vi "FipsAdjacent.vi"() -> (11 "Fips":i32[](array[numeric]))   [LabVIEW 2017] (continued)
08079\t\"Hinsdale County, CO\"\t08053\n\"Mineral County, CO\"\t08079\t\"Mineral County, CO\"\t08079\n\"Mineral County, CO\"\t08079\t\"Rio Grande County, CO\"\t08105\n\"Mineral County, CO\"\t08079\t\"Saguache County, CO\"\t08109\n\"Moffat County, CO\"\t08081\t\"Moffat County, CO\"\t08081\n\"Moffat County, CO\"\t08081\t\"Rio Blanco County, CO\"\t08103\n\"Moffat County, CO\"\t08081\t\"Routt County, CO\"\t08107\n\"Moffat County, CO\"\t08081\t\"Daggett County, UT\"\t49009\n\"Moffat County, CO\"\t08081\t\"Uintah County, UT\"\t49047\n\"Moffat County, CO\"\t08081\t\"Carbon County, WY\"\t56007\n\"Moffat County, CO\"\t08081\t\"Sweetwater County, WY\"\t56037\n\"Montezuma County, CO\"\t08083\t\"Apache County, AZ\"\t04001\n\"Montezuma County, CO\"\t08083\t\"Dolores County, CO\"\t08033\n\"Montezuma County, CO\"\t08083\t\"La Plata County, CO\"\t08067\n\"Montezuma County, CO\"\t08083\t\"Montezuma County, CO\"\t08083\n\"Montezuma County, CO\"\t08083\t\"San Juan County, CO\"\t08111\n\"Montezuma County, CO\"\t08083\t\"San Juan County, NM\"\t35045\n\"Montezuma County, CO\"\t08083\t\"San Juan County, UT\"\t49037\n\"Montrose County, CO\"\t08085\t\"Delta County, CO\"\t08029\n\"Montrose County, CO\"\t08085\t\"Gunnison County, CO\"\t08051\n\"Montrose County, CO\"\t08085\t\"Mesa County, CO\"\t08077\n\"Montrose County, CO\"\t08085\t\"Montrose County, CO\"\t08085\n\"Montrose County, CO\"\t08085\t\"Ouray County, CO\"\t08091\n\"Montrose County, CO\"\t08085\t\"San Miguel County, CO\"\t08113\n\"Montrose County, CO\"\t08085\t\"Grand County, UT\"\t49019\n\"Montrose County, CO\"\t08085\t\"San Juan County, UT\"\t49037\n\"Morgan County, CO\"\t08087\t\"Adams County, CO\"\t08001\n\"Morgan County, CO\"\t08087\t\"Logan County, CO\"\t08075\n\"Morgan County, CO\"\t08087\t\"Morgan County, CO\"\t08087\n\"Morgan County, CO\"\t08087\t\"Washington County, CO\"\t08121\n\"Morgan County, CO\"\t08087\t\"Weld County, CO\"\t08123\n\"Otero County, CO\"\t08089\t\"Bent County, CO\"\t08011\n\"Otero County, CO\"\t08089\t\"Crowley County, CO\"\t08025\n\"Otero County, CO\"\t08089\t\"Kiowa County, CO\"\t08061\n\"Otero County, CO\"\t08089\t\"Las Animas County, CO\"\t08071\n\"Otero County, CO\"\t08089\t\"Otero County, CO\"\t08089\n\"Otero County, CO\"\t08089\t\"Pueblo County, CO\"\t08101\n\"Ouray County, CO\"\t08091\t\"Gunnison County, CO\"\t08051\n\"Ouray County, CO\"\t08091\t\"Hinsdale County, CO\"\t08053\n\"Ouray County, CO\"\t08091\t\"Montrose County, CO\"\t08085\n\"Ouray County, CO\"\t08091\t\"Ouray County, CO\"\t08091\n\"Ouray County, CO\"\t08091\t\"San Juan County, CO\"\t08111\n\"Ouray County, CO\"\t08091\t\"San Miguel County, CO\"\t08113\n\"Park County, CO\"\t08093\t\"Chaffee County, CO\"\t08015\n\"Park County, CO\"\t08093\t\"Clear Creek County, CO\"\t08019\n\"Park County, CO\"\t08093\t\"Fremont County, CO\"\t08043\n\"Park County, CO\"\t08093\t\"Jefferson County, CO\"\t08059\n\"Park County, CO\"\t08093\t\"Lake County, CO\"\t08065\n\"Park County, CO\"\t08093\t\"Park County, CO\"\t08093\n\"Park County, CO\"\t08093\t\"Summit County, CO\"\t08117\n\"Park County, CO\"\t08093\t\"Teller County, CO\"\t08119\n\"Phillips County, CO\"\t08095\t\"Logan County, CO\"\t08075\n\"Phillips County, CO\"\t08095\t\"Phillips County, CO\"\t08095\n\"Phillips County, CO\"\t08095\t\"Sedgwick County, CO\"\t08115\n\"Phillips County, CO\"\t08095\t\"Yuma County, CO\"\t08125\n\"Phillips County, CO\"\t08095\t\"Chase County, NE\"\t31029\n\"Phillips County, CO\"\t08095\t\"Perkins County, NE\"\t31135\n\"Pitkin County, CO\"\t08097\t\"Chaffee County, CO\"\t08015\n\"Pitkin County, CO\"\t08097\t\"Eagle County, CO\"\t08037\n\"Pitkin County, CO\"\t08097\t\"Garfield County, CO\"\t08045\n\"Pitkin County, CO\"\t08097\t\"Gunnison County, CO\"\t08051\n\"Pitkin County, CO\"\t08097\t\"Lake County, CO\"\t08065\n\"Pitkin County, CO\"\t08097\t\"Mesa County, CO\"\t08077\n\"Pitkin County, CO\"\t08097\t\"Pitkin County, CO\"\t08097\n\"Prowers County, CO\"\t08099\t\"Baca County, CO\"\t08009\n\"Prowers County, CO\"\t08099\t\"Bent County, CO\"\t08011\n\"Prowers County, CO\"\t08099\t\"Kiowa County, CO\"\t08061\n\"Prowers County, CO\"\t08099\t\"Prowers County, CO\"\t08099\n\"Prowers County, CO\"\t08099\t\"Greeley County, KS\"\t20071\n\"Prowers County, CO\"\t08099\t\"Hamilton County, KS\"\t20075\n\"Prowers County, CO\"\t08099\t\"Stanton County, KS\"\t20187\n\"Pueblo County, CO\"\t08101\t\"Crowley County, CO\"\t08025\n\"Pueblo County, CO\"\t08101\t\"Custer County, CO\"\t08027\n\"Pueblo County, CO\"\t08101\t\"El Paso County, CO\"\t08041\n\"Pueblo County, CO\"\t08101\t\"Fremont County, CO\"\t08043\n\"Pueblo County, CO\"\t08101\t\"Huerfano County, CO\"\t08055\n\"Pueblo County, CO\"\t08101\t\"Las Animas County, CO\"\t08071\n\"Pueblo County, CO\"\t08101\t\"Lincoln County, CO\"\t08073\n\"Pueblo County, CO\"\t08101\t\"Otero County, CO\"\t08089\n\"Pueblo County, CO\"\t08101\t\"Pueblo County, CO\"\t08101\n\"Rio Blanco County, CO\"\t08103\t\"Garfield County, CO\"\t08045\n\"Rio Blanco County, CO\"\t08103\t\"Moffat County, CO\"\t08081\n\"Rio Blanco County, CO\"\t08103\t\"Rio Blanco County, CO\"\t08103\n\"Rio Blanco County, CO\"\t08103\t\"Routt County, CO\"\t08107\n\"Rio Blanco County, CO\"\t08103\t\"Uintah County, UT\"\t49047\n\"Rio Grande County, CO\"\t08105\t\"Alamosa County, CO\"\t08003\n\"Rio Grande County, CO\"\t08105\t\"Archuleta County, CO\"\t08007\n\"Rio Grande County, CO\"\t08105\t\"Conejos County, CO\"\t08021\n\"Rio Grande County, CO\"\t08105\t\"Mineral County, CO\"\t08079\n\"Rio Grande County, CO\"\t08105\t\"Rio Grande County, CO\"\t08105\n\"Rio Grande County, CO\"\t08105\t\"Saguache County, CO\"\t08109\n\"Routt County, CO\"\t08107\t\"Eagle County, CO\"\t08037\n\"Routt County, CO\"\t08107\t\"Garfield County, CO\"\t08045\n\"Routt County, CO\"\t08107\t\"Grand County, CO\"\t08049\n\"Routt County, CO\"\t08107\t\"Jackson County, CO\"\t08057\n\"Routt County, CO\"\t08107\t\"Moffat County, CO\"\t08081\n\"Routt County, CO\"\t08107\t\"Rio Blanco County, CO\"\t08103\n\"Routt County, CO\"\t08107\t\"Routt County, CO\"\t08107\n\"Routt County, CO\"\t08107\t\"Carbon County, WY\"\t56007\n\"Saguache County, CO\"\t08109\t\"Alamosa County, CO\"\t08003\n\"Saguache County, CO\"\t08109\t\"Chaffee County, CO\"\t08015\n\"Saguache County, CO\"\t08109\t\"Custer County, CO\"\t08027\n\"Saguache County, CO\"\t08109\t\"Fremont County, CO\"\t08043\n\"Saguache County, CO\"\t08109\t\"Gunnison County, CO\"\t08051\n\"Saguache County, CO\"\t08109\t\"Hinsdale County, CO\"\t08053\n\"Saguache County, CO\"\t08109\t\"Huerfano County, CO\"\t08055\n\"Saguache County, CO\"\t08109\t\"Mineral County, CO\"\t08079\n\"Saguache County, CO\"\t08109\t\"Rio Grande County, CO\"\t08105\n\"Saguache County, CO\"\t08109\t\"Saguache County, CO\"\t08109\n\"San Juan County, CO\"\t08111\t\"Dolores County, CO\"\t08033\n\"San Juan County, CO\"\t08111\t\"Hinsdale County, CO\"\t08053\n\"San Juan County, CO\"\t08111\t\"La Plata County, CO\"\t08067\n\"San Juan County, CO\"\t08111\t\"Montezuma County, CO\"\t08083\n\"San Juan County, CO\"\t08111\t\"Ouray County, CO\"\t08091\n\"San Juan County, CO\"\t08111\t\"San Juan County, CO\"\t08111\n\"San Juan County, CO\"\t08111\t\"San Miguel County, CO\"\t08113\n\"San Miguel County, CO\"\t08113\t\"Dolores County, CO\"\t08033\n\"San Miguel County, CO\"\t08113\t\"Montrose County, CO\"\t08085\n\"San Miguel County, CO\"\t08113\t\"Ouray County, CO\"\t08091\n\"San Miguel County, CO\"\t08113\t\"San Juan County, CO\"\t08111\n\"San Miguel County, CO\"\t08113\t\"San Miguel County, CO\"\t08113\n\"San Miguel County, CO\"\t08113\t\"San Juan County, UT\"\t49037\n\"Sedgwick County, CO\"\t08115\t\"Logan County, CO\"\t08075\n\"Sedgwick County, CO\"\t08115\t\"Phillips County, CO\"\t08095\n\"Sedgwick County, CO\"\t08115\t\"Sedgwick County, CO\"\t08115\n\"Sedgwick County, CO\"\t08115\t\"Cheyenne County, NE\"\t31033\n\"Sedgwick County, CO\"\t08115\t\"Deuel County, NE\"\t31049\n\"Sedgwick County, CO\"\t08115\t\"Perkins County, NE\"\t31135\n\"Summit County, CO\"\t08117\t\"Clear Creek County, CO\"\t08019\n\"Summit County, CO\"\t08117\t\"Eagle County, CO\"\t08037\n\"Summit County, CO\"\t08117\t\"Grand County, CO\"\t08049\n\"Summit County, CO\"\t08117\t\"Lake County, CO\"\t08065\n\"Summit County, CO\"\t08117\t\"Park County, CO\"\t08093\n\"Summit County, CO\"\t08117\t\"Summit County, CO\"\t08117\n\"Teller County, CO\"\t08119\t\"Douglas County, CO\"\t08035\n\"Teller County, CO\"\t08119\t\"El Paso County, CO\"\t08041\n\"Teller County, CO\"\t08119\t\"Fremont County, CO\"\t08043\n\"Teller County, CO\"\t08119\t\"Jefferson County, CO\"\t08059\n\"Teller County, CO\"\t08119\t\"Park County, CO\"\t08093\n\"Teller County, CO\"\t08119\t\"Teller County, CO\"\t08119\n\"Washington County, CO\"\t08121\t\"Adams County, CO\"\t08001\n\"Washington County, CO\"\t08121\t\"Arapahoe County, CO\"\t08005\n\"Washington County, CO\"\t08121\t\"Kit Carson County, CO\"\t08063\n\"Washington County, CO\"\t08121\t\"Lincoln County, CO\"\t08073\n\"Washington County, CO\"\t08121\t\"Logan County, CO\"\t08075\n\"Washington County, CO\"\t08121\t\"Morgan County, CO\"\t08087\n\"Washington County, CO\"\t08121\t\"Washington County, CO\"\t08121\n\"Washington County, CO\"\t08121\t\"Yuma County, CO\"\t08125\n\"Weld County, CO\"\t08123\t\"Adams County, CO\"\t08001\n\"Weld County, CO\"\t08123\t\"Boulder County, CO\"\t08013\n\"Weld County, CO\"\t08123\t\"Broomfield County, CO\"\t08014\n\"Weld County, CO\"\t08123\t\"Larimer County, CO\"\t08069\n\"Weld County, CO\"\t08123\t\"Logan County, CO\"\t08075\n\"Weld County, CO\"\t08123\t\"Morgan County, CO\"\t08087\n\"Weld County, CO\"\t08123\t\"Weld County, CO\"\t08123\n\"Weld County, CO\"\t08123\t\"Kimball County, NE\"\t31105\n\"Weld County, CO\"\t08123\t\"Laramie County, WY\"\t56021\n\"Yuma County, CO\"\t08125\t\"Kit Carson County, CO\"\t08063\n\"Yuma County, CO\"\t08125\t\"Logan County, CO\"\t08075\n\"Yuma County, CO\"\t08125\t\"Phillips County, CO\"\t08095\n\"Yuma County, CO\"\t08125\t\"Washington County, CO\"\t08121\n\"Yuma County, CO\"\t08125\t\"Yuma County, CO\"\t08125\n\"Yuma County, CO\"\t08125\t\"Cheyenne County, KS\"\t20023\n\"Yuma County, CO\"\t08125\t\"Chase County, NE\"\t31029\n\"Yuma County, CO\"\t08125\t\"Dundy County, NE\"\t31057\n\"Fairfield County, CT\"\t09001\t\"Fairfield County, CT\"\t09001\n\"Fairfield County, CT\"\t09001\t\"Litchfield County, CT\"\t09005\n\"Fairfield County, CT\"\t09001\t\"New Haven County, CT\"\t09009\n\"Fairfield County, CT\"\t09001\t\"Dutchess County, NY\"\t36027\n\"Fairfield County, CT\"\t09001\t\"Nassau County, NY\"\t36059\n\"Fairfield County, CT\"\t09001\t\"Putnam County, NY\"\t36079\n\"Fairfield County, CT\"\t09001\t\"Suffolk County, NY\"\t36103\n\"Fairfield County, CT\"\t09001\t\"Westchester County, NY\"\t36119\n\"Hartford County, CT\"\t09003\t\"Hartford County, CT\"\t09003\n\"Hartford County, CT\"\t09003\t\"Litchfield County, CT\"\t09005\n\"Hartford County, CT\"\t09003\t\"Middlesex County, CT\"\t09007\n\"Hartford County, CT\"\t09003\t\"New Haven County, CT\"\t09009\n\"Hartford County, CT\"\t09003\t\"New London County, CT\"\t09011\n\"Hartford County, CT\"\t09003\t\"Tolland County, CT\"\t09013\n\"Hartford County, CT\"\t09003\t\"Hampden County, MA\"\t25013\n\"Litchfield County, CT\"\t09005\t\"Fairfield County, CT\"\t09001\n\"Litchfield County, CT\"\t09005\t\"Hartford County, CT\"\t09003\n\"Litchfield County, CT\"\t09005\t\"Litchfield County, CT\"\t09005\n\"Litchfield County, CT\"\t09005\t\"New Haven County, CT\"\t09009\n\"Litchfield County, CT\"\t09005\t\"Berkshire County, MA\"\t25003\n\"Litchfield County, CT\"\t09005\t\"Hampden County, MA\"\t25013\n\"Litchfield County, CT\"\t09005\t\"Dutchess County, NY\"\t36027\n\"Middlesex County, CT\"\t09007\t\"Hartford County, CT\"\t09003\n\"Middlesex County, CT\"\t09007\t\"Middlesex County, CT\"\t09007\n\"Middlesex County, CT\"\t09007\t\"New Haven County, CT\"\t09009\n\"Middlesex County, CT\"\t09007\t\"New London County, CT\"\t09011\n\"Middlesex County, CT\"\t09007\t\"Suffolk County, NY\"\t36103\n\"New Haven County, CT\"\t09009\t\"Fairfield County, CT\"\t09001\n\"New Haven County, CT\"\t09009\t\"Hartford County, CT\"\t09003\n\"New Haven County, CT\"\t09009\t\"Litchfield County, CT\"\t09005\n\"New Haven County, CT\"\t09009\t\"Middlesex County, CT\"\t09007\n\"New Haven County, CT\"\t09009\t\"New Haven County, CT\"\t09009\n\"New Haven County, CT\"\t09009\t\"Suffolk County, NY\"\t36103\n\"New London County, CT\"\t09011\t\"Hartford County, CT\"\t09003\n\"New London County, CT\"\t09011\t\"Middlesex County, CT\"\t09007\n\"New London County, CT\"\t09011\t\"New London County, CT\"\t09011\n\"New London County, CT\"\t09011\t\"Tolland County, CT\"\t09013\n\"New London County, CT\"\t09011\t\"Windham County, CT\"\t09015\n\"New London County, CT\"\t09011\t\"Suffolk County, NY\"\t36103\n\"New London County, CT\"\t09011\t\"Kent County, RI\"\t44003\n\"New London County, CT\"\t09011\t\"Washington County, RI\"\t44009\n\"Tolland County, CT\"\t09013\t\"Hartford County, CT\"\t09003\n\"Tolland County, CT\"\t09013\t\"New London County, CT\"\t09011\n\"Tolland County, CT\"\t09013\t\"Tolland County, CT\"\t09013\n\"Tolland County, CT\"\t09013\t\"Windham County, CT\"\t09015\n\"Tolland County, CT\"\t09013\t\"Hampden County, MA\"\t25013\n\"Tolland County, CT\"\t09013\t\"Worcester County, MA\"\t25027\n\"Windham County, CT\"\t09015\t\"New London County, CT\"\t09011\n\"Windham County, CT\"\t09015\t\"Tolland County, CT\"\t09013\n\"Windham County, CT\"\t09015\t\"Windham County, CT\"\t09015\n\"Windham County, CT\"\t09015\t\"Worcester County, MA\"\t25027\n\"Windham County, CT\"\t09015\t\"Kent County, RI\"\t44003\n\"Windham County, CT\"\t09015\t\"Providence County, RI\"\t44007\n\"Kent County, DE\"\t10001\t\"Kent County, DE\"\t10001\n\"Kent County, DE\"\t10001\t\"New Castle County, DE\"\t10003\n\"Kent County, DE\"\t10001\t\"Sussex County, DE\"\t10005\n\"Kent County, DE\"\t10001\t\"Caroline County, MD\"\t24011\n\"Kent County, DE\"\t10001\t\"Kent County, MD\"\t24029\n\"Kent County, DE\"\t10001\t\"Queen Anne's County, MD\"\t24035\n\"Kent County, DE\"\t10001\t\"Cape May County, NJ\"\t34009\n\"Kent County, DE\"\t10001\t\"Cumberland County, NJ\"\t34011\n\"Kent County, DE\"\t10001\t\"Salem County, NJ\"\t34033\n\"New Castle County, DE\"\t10003\t\"Kent County, DE\"\t10001\n\"New Castle County, DE\"\t10003\t\"New Castle County, DE\"\t10003\n\"New Castle County, DE\"\t10003\t\"Cecil County, MD\"\t24015\n\"New Castle County, DE\"\t10003\t\"Kent County, MD\"\t24029\n\"New Castle County, DE\"\t10003\t\"Gloucester County, NJ\"\t34015\n\"New Castle County, DE\"\t10003\t\"Salem County, NJ\"\t34033\n\"New Castle County, DE\"\t10003\t\"Chester County, PA\"\t42029\n\"New Castle County, DE\"\t10003\t\"Delaware County, PA\"\t42045\n\"Sussex County, DE\"\t10005\t\"Kent County, DE\"\t10001\n\"Sussex County, DE\"\t10005\t\"Sussex County, DE\"\t10005\n\"Sussex County, DE\"\t10005\t\"Caroline County, MD\"\t24011\n\"Sussex County, DE\"\t10005\t\"Dorchester County, MD\"\t24019\n\"Sussex County, DE\"\t10005\t\"Wicomico County, MD\"\t24045\n\"Sussex County, DE\"\t10005\t\"Worcester County, MD\"\t24047\n\"Sussex County, DE\"\t10005\t\"Cape May County, NJ\"\t34009\n\"District of Columbia, DC\"\t11001\t\"District of Columbia, DC\"\t11001\n\"District of Columbia, DC\"\t11001\t\"Montgomery County, MD\"\t24031\n\"District of Columbia, DC\"\t11001\t\"Prince George's County, MD\"\t24033\n\"District of Columbia, DC\"\t11001\t\"Arlington County, VA\"\t51013\n\"District of Columbia, DC\"\t11001\t\"Fairfax County, VA\"\t51059\n\"District of Columbia, DC\"\t11001\t\"Alexandria city, VA\"\t51510\n\"Alachua County, FL\"\t12001\t\"Alachua County, FL\"\t12001\n\"Alachua County, FL\"\t12001\t\"Bradford County, FL\"\t12007\n\"Alachua County, FL\"\t12001\t\"Columbia County, FL\"\t12023\n\"Alachua County, FL\"\t12001\t\"Gilchrist County, FL\"\t12041\n\"Alachua County, FL\"\t12001\t\"Levy County, FL\"\t12075\n\"Alachua County, FL\"\t12001\t\"Marion County, FL\"\t12083\n\"Alachua County, FL\"\t12001\t\"Putnam County, FL\"\t12107\n\"Alachua County, FL\"\t12001\t\"Union County, FL\"\t12125\n\"Baker County, FL\"\t12003\t\"Baker County, FL\"\t12003\n\"Baker County, FL\"\t12003\t\"Bradford County, FL\"\t12007\n\"Baker County, FL\"\t12003\t\"Clay County, FL\"\t12019\n\"Baker County, FL\"\t12003\t\"Columbia County, FL\"\t12023\n\"Baker County, FL\"\t12003\t\"Duval County, FL\"\t12031\n\"Baker County, FL\"\t12003\t\"Nassau County, FL\"\t12089\n\"Baker County, FL\"\t12003\t\"Union County, FL\"\t12125\n\"Baker County, FL\"\t12003\t\"Charlton County, GA\"\t13049\n\"Baker County, FL\"\t12003\t\"Clinch County, GA\"\t13065\n\"Baker County, FL\"\t12003\t\"Ware County, GA\"\t13299\n\"Bay County, FL\"\t12005\t\"Bay County, FL\"\t12005\n\"Bay County, FL\"\t12005\t\"Calhoun County, FL\"\t12013\n\"Bay County, FL\"\t12005\t\"Gulf County, FL\"\t12045\n\"Bay County, FL\"\t12005\t\"Jackson County, FL\"\t12063\n\"Bay County, FL\"\t12005\t\"Walton County, FL\"\t12131\n\"Bay County, FL\"\t12005\t\"Washington County, FL\"\t12133\n\"Bradford County, FL\"\t12007\t\"Alachua County, FL\"\t12001\n\"Bradford County, FL\"\t12007\t\"Baker County, FL\"\t12003\n\"Bradford County, FL\"\t12007\t\"Bradford County, FL\"\t12007\n\"Bradford County, FL\"\t12007\t\"Clay County, FL\"\t12019\n\"Bradford County, FL\"\t12007\t\"Putnam County, FL\"\t12107\n\"Bradford County, FL\"\t12007\t\"Union County, FL\"\t12125\n\"Brevard County, FL\"\t12009\t\"Brevard County, FL\"\t12009\n\"Brevard County, FL\"\t12009\t\"Indian River County, FL\"\t12061\n\"Brevard County, FL\"\t12009\t\"Orange County, FL\"\t12095\n\"Brevard County, FL\"\t12009\t\"Osceola County, FL\"\t12097\n\"Brevard County, FL\"\t12009\t\"Seminole County, FL\"\t12117\n\"Brevard County, FL\"\t12009\t\"Volusia County, FL\"\t12127\n\"Broward County, FL\"\t12011\t\"Broward County, FL\"\t12011\n\"Broward County, FL\"\t12011\t\"Collier County, FL\"\t12021\n\"Broward County, FL\"\t12011\t\"Hendry County, FL\"\t12051\n\"Broward County, FL\"\t12011\t\"Miami-Dade County, FL\"\t12086\n\"Broward County, FL\"\t12011\t\"Palm Beach County, FL\"\t12099\n\"Calhoun County, FL\"\t12013\t\"Bay County, FL\"\t12005\n\"Calhoun County, FL\"\t12013\t\"Calhoun County, FL\"\t12013\n\"Calhoun County, FL\"\t12013\t\"Gadsden County, FL\"\t12039\n\"Calhoun County, FL\"\t12013\t\"Gulf County, FL\"\t12045\n\"Calhoun County, FL\"\t12013\t\"Jackson County, FL\"\t12063\n\"Calhoun County, FL\"\t12013\t\"Liberty County, FL\"\t12077\n\"Charlotte County, FL\"\t12015\t\"Charlotte County, FL\"\t12015\n\"Charlotte County, FL\"\t12015\t\"DeSoto County, FL\"\t12027\n\"Charlotte County, FL\"\t12015\t\"Glades County, FL\"\t12043\n\"Charlotte County, FL\"\t12015\t\"Hendry County, FL\"\t12051\n\"Charlotte County, FL\"\t12015\t\"Highlands County, FL\"\t12055\n\"Charlotte County, FL\"\t12015\t\"Lee County, FL\"\t12071\n\"Charlotte County, FL\"\t12015\t\"Sarasota County, FL\"\t12115\n\"Citrus County, FL\"\t12017\t\"Citrus County, FL\"\t12017\n\"Citrus County, FL\"\t12017\t\"Hernando County, FL\"\t12053\n\"Citrus County, FL\"\t12017\t\"Levy County, FL\"\t12075\n\"Citrus County, FL\"\t12017\t\"Marion County, FL\"\t12083\n\"Citrus County, FL\"\t12017\t\"Sumter County, FL\"\t12119\n\"Clay County, FL\"\t12019\t\"Baker County, FL\"\t12003\n\"Clay County, FL\"\t12019\t\"Bradford County, FL\"\t12007\n\"Clay County, FL\"\t12019\t\"Clay County, FL\"\t12019\n\"Clay County, FL\"\t12019\t\"Duval County, FL\"\t12031\n\"Clay County, FL\"\t12019\t\"Putnam County, FL\"\t12107\n\"Clay County, FL\"\t12019\t\"St. Johns County, FL\"\t12109\n\"Collier County, FL\"\t12021\t\"Broward County, FL\"\t12011\n\"Collier County, FL\"\t12021\t\"Collier County, FL\"\t12021\n\"Collier County, FL\"\t12021\t\"Hendry County, FL\"\t12051\n\"Collier County, FL\"\t12021\t\"Lee County, FL\"\t12071\n\"Collier County, FL\"\t12021\t\"Miami-Dade County, FL\"\t12086\n\"Collier County, FL\"\t12021\t\"Monroe County, FL\"\t12087\n\"Columbia County, FL\"\t12023\t\"Alachua County, FL\"\t12001\n\"Columbia County, FL\"\t12023\t\"Baker County, FL\"\t12003\n\"Columbia County, FL\"\t12023\t\"Columbia County, FL\"\t12023\n\"Columbia County, FL\"\t12023\t\"Gilchrist County, FL\"\t12041\n\"Columbia County, FL\"\t12023\t\"Hamilton County, FL\"\t12047\n\"Columbia County, FL\"\t12023\t\"Suwannee County, FL\"\t12121\n\"Columbia County, FL\"\t12023\t\"Union County, FL\"\t12125\n\"Columbia County, FL\"\t12023\t\"Clinch County, GA\"\t13065\n\"Columbia County, FL\"\t12023\t\"Echols County, GA\"\t13101\n\"DeSoto County, FL\"\t12027\t\"Charlotte County, FL\"\t12015\n\"DeSoto County, FL\"\t12027\t\"DeSoto County, FL\"\t12027\n\"DeSoto County, FL\"\t12027\t\"Glades County, FL\"\t12043\n\"DeSoto County, FL\"\t12027\t\"Hardee County, FL\"\t12049\n\"DeSoto County, FL\"\t12027\t\"Highlands County, FL\"\t12055\n\"DeSoto County, FL\"\t12027\t\"Manatee County, FL\"\t12081\n\"DeSoto County, FL\"\t12027\t\"Sarasota County, FL\"\t12115\n\"Dixie County, FL\"\t12029\t\"Dixie County, FL\"\t12029\n\"Dixie County, FL\"\t12029\t\"Gilchrist County, FL\"\t12041\n\"Dixie County, FL\"\t12029\t\"Lafayette County, FL\"\t12067\n\"Dixie County, FL\"\t12029\t\"Levy County, FL\"\t12075\n\"Dixie County, FL\"\t12029\t\"Taylor County, FL\"\t12123\n\"Duval County, FL\"\t12031\t\"Baker County, FL\"\t12003\n\"Duval County, FL\"\t12031\t\"Clay County, FL\"\t12019\n\"Duval County, FL\"\t12031\t\"Duval County, FL\"\t12031\n\"Duval County, FL\"\t12031\t\"Nassau County, FL\"\t12089\n\"Duval County, FL\"\t12031\t\"St. Johns County, FL\"\t12109\n\"Escambia County, FL\"\t12033\t\"Baldwin County, AL\"\t01003\n\"Escambia County, FL\"\t12033\t\"Escambia County, AL\"\t01053\n\"Escambia County, FL\"\t12033\t\"Escambia County, FL\"\t12033\n\"Escambia County, FL\"\t12033\t\"Santa Rosa County, FL\"\t12113\n\"Flagler County, FL\"\t12035\t\"Flagler County, FL\"\t12035\n\"Flagler County, FL\"\t12035\t\"Putnam County, FL\"\t12107\n\"Flagler County, FL\"\t12035\t\"St. Johns County, FL\"\t12109\n\"Flagler County, FL\"\t12035\t\"Volusia County, FL\"\t12127\n\"Franklin County, FL\"\t12037\t\"Franklin County, FL\"\t12037\n\"Franklin County, FL\"\t12037\t\"Gulf County, FL\"\t12045\n\"Franklin County, FL\"\t12037\t\"Liberty County, FL\"\t12077\n\"Franklin County, FL\"\t12037\t\"Wakulla County, FL\"\t12129\n\"Gadsden County, FL\"\t12039\t\"Calhoun County, FL\"\t12013\n\"Gadsden County, FL\"\t12039\t\"Gadsden County, FL\"\t12039\n\"Gadsden County, FL\"\t12039\t\"Jackson County, FL\"\t12063\n\"Gadsden County, FL\"\t12039\t\"Leon County, FL\"\t12073\n\"Gadsden County, FL\"\t12039\t\"Liberty County, FL\"\t12077\n\"Gadsden County, FL\"\t12039\t\"Decatur County, GA\"\t13087\n\"Gadsden County, FL\"\t12039\t\"Grady County, GA\"\t13131\n\"Gadsden County, FL\"\t12039\t\"Seminole County, GA\"\t13253\n\"Gilchrist County, FL\"\t12041\t\"Alachua County, FL\"\t12001\n\"Gilchrist County, FL\"\t12041\t\"Columbia County, FL\"\t12023\n\"Gilchrist County, FL\"\t12041\t\"Dixie County, FL\"\t12029\n\"Gilchrist County, FL\"\t12041\t\"Gilchrist County, FL\"\t12041\n\"Gilchrist County, FL\"\t12041\t\"Lafayette County, FL\"\t12067\n\"Gilchrist County, FL\"\t12041\t\"Levy County, FL\"\t12075\n\"Gilchrist County, FL\"\t12041\t\"Suwannee County, FL\"\t12121\n\"Glades County, FL\"\t12043\t\"Charlotte County, FL\"\t12015\n\"Glades County, FL\"\t12043\t\"DeSoto County, FL\"\t12027\n\"Glades County, FL\"\t12043\t\"Glades County, FL\"\t12043\n\"Glades County, FL\"\t12043\t\"Hendry County, FL\"\t12051\n\"Glades County, FL\"\t12043\t\"Highlands County, FL\"\t12055\n\"Glades County, FL\"\t12043\t\"Lee County, FL\"\t12071\n\"Glades County, FL\"\t12043\t\"Martin County, FL\"\t12085\n\"Glades County, FL\"\t12043\t\"Okeechobee County, FL\"\t12093\n\"Glades County, FL\"\t12043\t\"Palm Beach County, FL\"\t12099\n\"Gulf County, FL\"\t12045\t\"Bay County, FL\"\t12005\n\"Gulf County, FL\"\t12045\t\"Calhoun County, FL\"\t12013\n\"Gulf County, FL\"\t12045\t\"Franklin County, FL\"\t12037\n\"Gulf County, FL\"\t12045\t\"Gulf County, FL\"\t12045\n\"Gulf County, FL\"\t12045\t\"Liberty County, FL\"\t12077\n\"Hamilton County, FL\"\t12047\t\"Columbia County, FL\"\t12023\n\"Hamilton County, FL\"\t12047\t\"Hamilton County, FL\"\t12047\n\"Hamilton County, FL\"\t12047\t\"Madison County, FL\"\t12079\n\"Hamilton County, FL\"\t12047\t\"Suwannee County, FL\"\t12121\n\"Hamilton County, FL\"\t12047\t\"Brooks County, GA\"\t13027\n\"Hamilton County, FL\"\t12047\t\"Echols County, GA\"\t13101\n\"Hamilton County, FL\"\t12047\t\"Lowndes County, GA\"\t13185\n\"Hardee County, FL\"\t12049\t\"DeSoto County, FL\"\t12027\n\"Hardee County, FL\"\t12049\t\"Hardee County, FL\"\t12049\n\"Hardee County, FL\"\t12049\t\"Highlands County, FL\"\t12055\n\"Hardee County, FL\"\t12049\t\"Hillsborough County, FL\"\t12057\n\"Hardee County, FL\"\t12049\t\"Manatee County, FL\"\t12081\n\"Hardee County, FL\"\t12049\t\"Polk County, FL\"\t12105\n\"Hendry County, FL\"\t12051\t\"Broward County, FL\"\t12011\n\"Hendry County, FL\"\t12051\t\"Charlotte County, FL\"\t12015\n\"Hendry County, FL\"\t12051\t\"Collier County, FL\"\t12021\n\"Hendry County, FL\"\t12051\t\"Glades County, FL\"\t12043\n\"Hendry County, FL\"\t12051\t\"Hendry County, FL\"\t12051\n\"Hendry County, FL\"\t12051\t\"Lee County, FL\"\t12071\n\"Hendry County, FL\"\t12051\t\"Martin County, FL\"\t12085\n\"Hendry County, FL\"\t12051\t\"Okeechobee County, FL\"\t12093\n\"Hendry County, FL\"\t12051\t\"Palm Beach County, FL\"\t12099\n\"Hernando County, FL\"\t12053\t\"Citrus County, FL\"\t12017\n\"Hernando County, FL\"\t12053\t\"Hernando County, FL\"\t12053\n\"Hernando County, FL\"\t12053\t\"Pasco County, FL\"\t12101\n\"Hernando County, FL\"\t12053\t\"Sumter County, FL\"\t12119\n\"Highlands County, FL\"\t12055\t\"Charlotte County, FL\"\t12015\n\"Highlands County, FL\"\t12055\t\"DeSoto County, FL\"\t12027\n\"Highlands County, FL\"\t12055\t\"Glades County, FL\"\t12043\n\"Highlands County, FL\"\t12055\t\"Hardee County, FL\"\t12049\n\"Highlands County, FL\"\t12055\t\"Highlands County, FL\"\t12055\n\"Highlands County, FL\"\t12055\t\"Okeechobee County, FL\"\t12093\n\"Highlands County, FL\"\t12055\t\"Osceola County, FL\"\t12097\n\"Highlands County, FL\"\t12055\t\"Polk County, FL\"\t12105\n\"Hillsborough County, FL\"\t12057\t\"Hardee County, FL\"\t12049\n\"Hillsborough County, FL\"\t12057\t\"Hillsborough County, FL\"\t12057\n\"Hillsborough County, FL\"\t12057\t\"Manatee County, FL\"\t12081\n\"Hillsborough County, FL\"\t12057\t\"Pasco County, FL\"\t12101\n\"Hillsborough County, FL\"\t12057\t\"Pinellas County, FL\"\t12103\n\"Hillsborough County, FL\"\t12057\t\"Polk County, FL\"\t12105\n\"Holmes County, FL\"\t12059\t\"Geneva County, AL\"\t01061\n\"Holmes County, FL\"\t12059\t\"Holmes County, FL\"\t12059\n\"Holmes County, FL\"\t12059\t\"Jackson County, FL\"\t12063\n\"Holmes County, FL\"\t12059\t\"Walton County, FL\"\t12131\n\"Holmes County, FL\"\t12059\t\"Washington County, FL\"\t12133\n\"Indian River County, FL\"\t12061\t\"Brevard County, FL\"\t12009\n\"Indian River County, FL\"\t12061\t\"Indian River County, FL\"\t12061\n\"Indian River County, FL\"\t12061\t\"Okeechobee County, FL\"\t12093\n\"Indian River County, FL\"\t12061\t\"Osceola County, FL\"\t12097\n\"Indian River County, FL\"\t12061\t\"St. Lucie County, FL\"\t12111\n\"Jackson County, FL\"\t12063\t\"Geneva County, AL\"\t01061\n\"Jackson County, FL\"\t12063\t\"Houston County, AL\"\t01069\n\"Jackson County, FL\"\t12063\t\"Bay County, FL\"\t12005\n\"Jackson County, FL\"\t12063\t\"Calhoun County, FL\"\t12013\n\"Jackson County, FL\"\t12063\t\"Gadsden County, FL\"\t12039\n\"Jackson County, FL\"\t12063\t\"Holmes County, FL\"\t12059\n\"Jackson County, FL\"\t12063\t\"Jackson County, FL\"\t12063\n\"Jackson County, FL\"\t12063\t\"Liberty County, FL\"\t12077\n\"Jackson County, FL\"\t12063\t\"Washington County, FL\"\t12133\n\"Jackson County, FL\"\t12063\t\"Seminole County, GA\"\t13253\n\"Jefferson County, FL\"\t12065\t\"Jefferson County, FL\"\t12065\n\"Jefferson County, FL\"\t12065\t\"Leon County, FL\"\t12073\n\"Jefferson County, FL\"\t12065\t\"Madison County, FL\"\t12079\n\"Jefferson County, FL\"\t12065\t\"Taylor County, FL\"\t12123\n\"Jefferson County, FL\"\t12065\t\"Wakulla County, FL\"\t12129\n\"Jefferson County, FL\"\t12065\t\"Brooks County, GA\"\t13027\n\"Jefferson County, FL\"\t12065\t\"Thomas County, GA\"\t13275\n\"Lafayette County, FL\"\t12067\t\"Dixie County, FL\"\t12029\n\"Lafayette County, FL\"\t12067\t\"Gilchrist County, FL\"\t12041\n\"Lafayette County, FL\"\t12067\t\"Lafayette County, FL\"\t12067\n\"Lafayette County, FL\"\t12067\t\"Madison County, FL\"\t12079\n\"Lafayette County, FL\"\t12067\t\"Suwannee County, FL\"\t12121\n\"Lafayette County, FL\"\t12067\t\"Taylor County, FL\"\t12123\n\"Lake County, FL\"\t12069\t\"Lake County, FL\"\t12069\n\"Lake County, FL\"\t12069\t\"Marion County, FL\"\t12083\n\"Lake County, FL\"\t12069\t\"Orange County, FL\"\t12095\n\"Lake County, FL\"\t12069\t\"Osceola County, FL\"\t12097\n\"Lake County, FL\"\t12069\t\"Polk County, FL\"\t12105\n\"Lake County, FL\"\t12069\t\"Seminole County, FL\"\t12117\n\"Lake County, FL\"\t12069\t\"Sumter County, FL\"\t12119\n\"Lake County, FL\"\t12069\t\"Volusia County, FL\"\t12127\n\"Lee County, FL\"\t12071\t\"Charlotte County, FL\"\t12015\n\"Lee County, FL\"\t12071\t\"Collier County, FL\"\t12021\n\"Lee County, FL\"\t12071\t\"Glades County, FL\"\t12043\n\"Lee County, FL\"\t12071\t\"Hendry County, FL\"\t12051\n\"Lee County, FL\"\t12071\t\"Lee County, FL\"\t12071\n\"Leon County, FL\"\t12073\t\"Gadsden County, FL\"\t12039\n\"Leon County, FL\"\t12073\t\"Jefferson County, FL\"\t12065\n\"Leon County, FL\"\t12073\t\"Leon County, FL\"\t12073\n\"Leon County, FL\"\t12073\t\"Liberty County, FL\"\t12077\n\"Leon County, FL\"\t12073\t\"Wakulla County, FL\"\t12129\n\"Leon County, FL\"\t12073\t\"Grady County, GA\"\t13131\n\"Leon County, FL\"\t12073\t\"Thomas County, GA\"\t13275\n\"Levy County, FL\"\t12075\t\"Alachua County, FL\"\t12001\n\"Levy County, FL\"\t12075\t\"Citrus County, FL\"\t12017\n\"Levy County, FL\"\t12075\t\"Dixie County, FL\"\t12029\n\"Levy County, FL\"\t12075\t\"Gilchrist County, FL\"\t12041\n\"Levy County, FL\"\t12075\t\"Levy County, FL\"\t12075\n\"Levy County, FL\"\t12075\t\"Marion County, FL\"\t12083\n\"Liberty County, FL\"\t12077\t\"Calhoun County, FL\"\t12013\n\"Liberty County, FL\"\t12077\t\"Franklin County, FL\"\t12037\n\"Liberty County, FL\"\t12077\t\"Gadsden County, FL\"\t12039\n\"Liberty County, FL\"\t12077\t\"Gulf County, FL\"\t12045\n\"Liberty County, FL\"\t12077\t\"Jackson County, FL\"\t12063\n\"Liberty County, FL\"\t12077\t\"Leon County, FL\"\t12073\n\"Liberty County, FL\"\t12077\t\"Liberty County, FL\"\t12077\n\"Liberty County, FL\"\t12077\t\"Wakulla County, FL\"\t12129\n\"Madison County, FL\"\t12079\t\"Hamilton County, FL\"\t12047\n\"Madison County, FL\"\t12079\t\"Jefferson County, FL\"\t12065\n\"Madison County, FL\"\t12079\t\"Lafayette County, FL\"\t12067\n\"Madison County, FL\"\t12079\t\"Madison County, FL\"\t12079\n\"Madison County, FL\"\t12079\t\"Suwannee County, FL\"\t12121\n\"Madison County, FL\"\t12079\t\"Taylor County, FL\"\t12123\n\"Madison County, FL\"\t12079\t\"Brooks County, GA\"\t13027\n\"Madison County, FL\"\t12079\t\"Lowndes County, GA\"\t13185\n\"Manatee County, FL\"\t12081\t\"DeSoto County, FL\"\t12027\n\"Manatee County, FL\"\t12081\t\"Hardee County, FL\"\t12049\n\"Manatee County, FL\"\t12081\t\"Hillsborough County, FL\"\t12057\n\"Manatee County, FL\"\t12081\t\"Manatee County, FL\"\t12081\n\"Manatee County, FL\"\t12081\t\"Polk County, FL\"\t12105\n\"Manatee County, FL\"\t12081\t\"Sarasota County, FL\"\t12115\n\"Marion County, FL\"\t12083\t\"Alachua County, FL\"\t12001\n\"Marion County, FL\"\t12083\t\"Citrus County, FL\"\t12017\n\"Marion County, FL\"\t12083\t\"Lake County, FL\"\t12069\n\"Marion County, FL\"\t12083\t\"Levy County, FL\"\t12075\n\"Marion County, FL\"\t12083\t\"Marion County, FL\"\t12083\n\"Marion County, FL\"\t12083\t\"Putnam County, FL\"\t12107\n\"Marion County, FL\"\t12083\t\"Sumter County, FL\"\t12119\n\"Marion County, FL\"\t12083\t\"Volusia County, FL\"\t12127\n\"Martin County, FL\"\t12085\t\"Glades County, FL\"\t12043\n\"Martin County, FL\"\t12085\t\"Hendry County, FL\"\t12051\n\"Martin County, FL\"\t12085\t\"Martin County, FL\"\t12085\n\"Martin County, FL\"\t12085\t\"Okeechobee County, FL\"\t12093\n\"Martin County, FL\"\t12085\t\"Palm Beach County, FL\"\t12099\n\"Martin County, FL\"\t12085\t\"St. Lucie County, FL\"\t12111\n\"Miami-Dade County, FL\"\t12086\t\"Broward County, FL\"\t12011\n\"Miami-Dade County, FL\"\t12086\t\"Collier County, FL\"\t12021\n\"Miami-Dade County, FL\"\t12086\t\"Miami-Dade County, FL\"\t12086\n\"Miami-Dade County, FL\"\t12086\t\"Monroe County, FL\"\t12087\n\"Monroe County, FL\"\t12087\t\"Collier County, FL\"\t12021\n\"Monroe County, FL\"\t12087\t\"Miami-Dade County, FL\"\t12086\n\"Monroe County, FL\"\t12087\t\"Monroe County, FL\"\t12087\n\"Nassau County, FL\"\t12089\t\"Baker County, FL\"\t12003\n\"Nassau County, FL\"\t12089\t\"Duval County, FL\"\t12031\n\"Nassau County, FL\"\t12089\t\"Nassau County, FL\"\t12089\n\"Nassau County, FL\"\t12089\t\"Camden County, GA\"\t13039\n\"Nassau County, FL\"\t12089\t\"Charlton County, GA\"\t13049\n\"Okaloosa County, FL\"\t12091\t\"Covington County, AL\"\t01039\n\"Okaloosa County, FL\"\t12091\t\"Escambia County, AL\"\t01053\n\"Okaloosa County, FL\"\t12091\t\"Okaloosa County, FL\"\t12091\n\"Okaloosa County, FL\"\t12091\t\"Santa Rosa County, FL\"\t12113\n\"Okaloosa County, FL\"\t12091\t\"Walton County, FL\"\t12131\n\"Okeechobee County, FL\"\t12093\t\"Glades County, FL\"\t12043\n\"Okeechobee County, FL\"\t12093\t\"Hendry County, FL\"\t12051\n\"Okeechobee County, FL\"\t12093\t\"Highlands County, FL\"\t12055\n\"Okeechobee County, FL\"\t12093\t\"Indian River County, FL\"\t12061\n\"Okeechobee County, FL\"\t12093\t\"Martin County, FL\"\t12085\n\"Okeechobee County, FL\"\t12093\t\"Okeechobee County, FL\"\t12093\n\"Okeechobee County, FL\"\t12093\t\"Osceola County, FL\"\t12097\n\"Okeechobee County, FL\"\t12093\t\"Palm Beach County, FL\"\t12099\n\"Okeechobee County, FL\"\t12093\t\"Polk County, FL\"\t12105\n\"Okeechobee County, FL\"\t12093\t\"St. Lucie County, FL\"\t12111\n\"Orange County, FL\"\t12095\t\"Brevard County, FL\"\t12009\n\"Orange County, FL\"\t12095\t\"Lake County, FL\"\t12069\n\"Orange County, FL\"\t12095\t\"Orange County, FL\"\t12095\n\"Orange County, FL\"\t12095\t\"Osceola County, FL\"\t12097\n\"Orange County, FL\"\t12095\t\"Polk County, FL\"\t12105\n\"Orange County, FL\"\t12095\t\"Seminole County, FL\"\t12117\n\"Orange County, FL\"\t12095\t\"Volusia County, FL\"\t12127\n\"Osceola County, FL\"\t12097\t\"Brevard County, FL\"\t12009\n\"Osceola County, FL\"\t12097\t\"Highlands County, FL\"\t12055\n\"Osceola County, FL\"\t12097\t\"Indian River County, FL\"\t12061\n\"Osceola County, FL\"\t12097\t\"Lake County, FL\"\t12069\n\"Osceola County, FL\"\t12097\t\"Okeechobee County, FL\"\t12093\n\"Osceola County, FL\"\t12097\t\"Orange County, FL\"\t12095\n\"Osceola County, FL\"\t12097\t\"Osceola County, FL\"\t12097\n\"Osceola County, FL\"\t12097\t\"Polk County, FL\"\t12105\n\"Palm Beach County, FL\"\t12099\t\"Broward County, FL\"\t12011\n\"Palm Beach County, FL\"\t12099\t\"Glades County, FL\"\t12043\n\"Palm Beach County, FL\"\t12099\t\"Hendry County, FL\"\t12051\n\"Palm Beach County, FL\"\t12099\t\"Martin County, FL\"\t12085\n\"Palm Beach County, FL\"\t12099\t\"Okeechobee County, FL\"\t12093\n\"Palm Beach County, FL\"\t12099\t\"Palm Beach County, FL\"\t12099\n\"Pasco County, FL\"\t12101\t\"Hernando County, FL\"\t12053\n\"Pasco County, FL\"\t12101\t\"Hillsborough County, FL\"\t12057\n\"Pasco County, FL\"\t12101\t\"Pasco County, FL\"\t12101\n\"Pasco County, FL\"\t12101\t\"Pinellas County, FL\"\t12103\n\"Pasco County, FL\"\t12101\t\"Polk County, FL\"\t12105\n\"Pasco County, FL\"\t12101\t\"Sumter County, FL\"\t12119\n\"Pinellas County, FL\"\t12103\t\"Hillsborough County, FL\"\t12057\n\"Pinellas County, FL\"\t12103\t\"Pasco County, FL\"\t12101\n\"Pinellas County, FL\"\t12103\t\"Pinellas County, FL\"\t12103\n\"Polk County, FL\"\t12105\t\"Hardee County, FL\"\t12049\n\"Polk County, FL\"\t12105\t\"Highlands County, FL\"\t12055\n\"Polk County, FL\"\t12105\t\"Hillsborough County, FL\"\t12057\n\"Polk County, FL\"\t12105\t\"Lake County, FL\"\t12069\n\"Polk County, FL\"\t12105\t\"Manatee County, FL\"\t12081\n\"Polk County, FL\"\t12105\t\"Okeechobee County, FL\"\t12093\n\"Polk County, FL\"\t12105\t\"Orange County, FL\"\t12095\n\"Polk County, FL\"\t12105\t\"Osceola County, FL\"\t12097\n\"Polk County, FL\"\t12105\t\"Pasco County, FL\"\t12101\n\"Polk County, FL\"\t12105\t\"Polk County, FL\"\t12105\n\"Polk County, FL\"\t12105\t\"Sumter County, FL\"\t12119\n\"Putnam County, FL\"\t12107\t\"Alachua County, FL\"\t12001\n\"Putnam County, FL\"\t12107\t\"Bradford County, FL\"\t12007\n\"Putnam County, FL\"\t12107\t\"Clay County, FL\"\t12019\n\"Putnam County, FL\"\t12107\t\"Flagler County, FL\"\t12035\n\"Putnam County, FL\"\t12107\t\"Marion County, FL\"\t12083\n\"Putnam County, FL\"\t12107\t\"Putnam County, FL\"\t12107\n\"Putnam County, FL\"\t12107\t\"St. Johns County, FL\"\t12109\n\"Putnam County, FL\"\t12107\t\"Volusia County, FL\"\t12127\n\"St. Johns County, FL\"\t12109\t\"Clay County, FL\"\t12019\n\"St. Johns County, FL\"\t12109\t\"Duval County, FL\"\t12031\n\"St. Johns County, FL\"\t12109\t\"Flagler County, FL\"\t12035\n\"St. Johns County, FL\"\t12109\t\"Putnam County, FL\"\t12107\n\"St. Johns County, FL\"\t12109\t\"St. Johns County, FL\"\t12109\n\"St. Lucie County, FL\"\t12111\t\"Indian River County, FL\"\t12061\n\"St. Lucie County, FL\"\t12111\t\"Martin County, FL\"\t12085\n\"St. Lucie County, FL\"\t12111\t\"Okeechobee County, FL\"\t12093\n\"St. Lucie County, FL\"\t12111\t\"St. Lucie County, FL\"\t12111\n\"Santa Rosa County, FL\"\t12113\t\"Escambia County, AL\"\t01053\n\"Santa Rosa County, FL\"\t12113\t\"Escambia County, FL\"\t12033\n\"Santa Rosa County, FL\"\t12113\t\"Okaloosa County, FL\"\t12091\n\"Santa Rosa County, FL\"\t12113\t\"Santa Rosa County, FL\"\t12113\n\"Sarasota County, FL\"\t12115\t\"Charlotte County, FL\"\t12015\n\"Sarasota County, FL\"\t12115\t\"DeSoto County, FL\"\t12027\n\"Sarasota County, FL\"\t12115\t\"Manatee County, FL\"\t12081\n\"Sarasota County, FL\"\t12115\t\"Sarasota County, FL\"\t12115\n\"Seminole County, FL\"\t12117\t\"Brevard County, FL\"\t12009\n\"Seminole County, FL\"\t12117\t\"Lake County, FL\"\t12069\n\"Seminole County, FL\"\t12117\t\"Orange County, FL\"\t12095\n\"Seminole County, FL\"\t12117\t\"Seminole County, FL\"\t12117\n\"Seminole County, FL\"\t12117\t\"Volusia County, FL\"\t12127\n\"Sumter County, FL\"\t12119\t\"Citrus County, FL\"\t12017\n\"Sumter County, FL\"\t12119\t\"Hernando County, FL\"\t12053\n\"Sumter County, FL\"\t12119\t\"Lake County, FL\"\t12069\n\"Sumter County, FL\"\t12119\t\"Marion County, FL\"\t12083\n\"Sumter County, FL\"\t12119\t\"Pasco County, FL\"\t12101\n\"Sumter County, FL\"\t12119\t\"Polk County, FL\"\t12105\n\"Sumter County, FL\"\t12119\t\"Sumter County, FL\"\t12119\n\"Suwannee County, FL\"\t12121\t\"Columbia County, FL\"\t12023\n\"Suwannee County, FL\"\t12121\t\"Gilchrist County, FL\"\t12041\n\"Suwannee County, FL\"\t12121\t\"Hamilton County, FL\"\t12047\n\"Suwannee County, FL\"\t12121\t\"Lafayette County, FL\"\t12067\n\"Suwannee County, FL\"\t12121\t\"Madison County, FL\"\t12079\n\"Suwannee County, FL\"\t12121\t\"Suwannee County, FL\"\t12121\n\"Taylor County, FL\"\t12123\t\"Dixie County, FL\"\t12029\n\"Taylor County, FL\"\t12123\t\"Jefferson County, FL\"\t12065\n\"Taylor County, FL\"\t12123\t\"Lafayette County, FL\"\t12067\n\"Taylor County, FL\"\t12123\t\"Madison County, FL\"\t12079\n\"Taylor County, FL\"\t12123\t\"Taylor County, FL\"\t12123\n\"Union County, FL\"\t12125\t\"Alachua County, FL\"\t12001\n\"Union County, FL\"\t12125\t\"Baker County, FL\"\t12003\n\"Union County, FL\"\t12125\t\"Bradford County, FL\"\t12007\n\"Union County, FL\"\t12125\t\"Columbia County, FL\"\t12023\n\"Union County, FL\"\t12125\t\"Union County, FL\"\t12125\n\"Volusia County, FL\"\t12127\t\"Brevard County, FL\"\t12009\n\"Volusia County, FL\"\t12127\t\"Flagler County, FL\"\t12035\n\"Volusia County, FL\"\t12127\t
